vi "Main.vi"() -> ()   [LabVIEW 2025]
panel:
  out "Available Cash":dbl
  out "Password Exist?":bool
  in  "Input":string
  in  "Exit":bool
  in  "Fast Cash (50)":bool
  in  "Deposit":bool
  in  "Withdraw":bool
  in  "Login":bool
  out "ATM window":string
  in  "Tab Control":enum32{"ATM"}(tab)
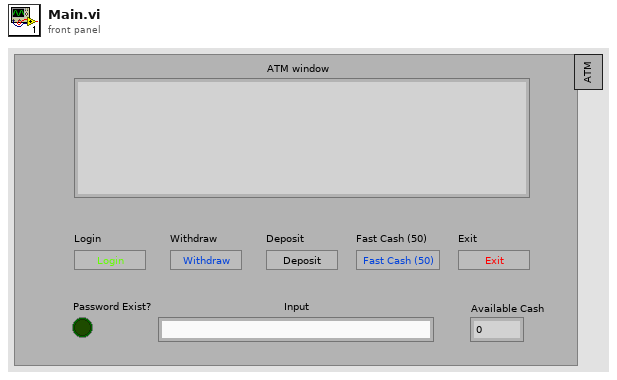
[diagram p1: front panel]
types:
  T1 = cluster{"Data":string[][], "User_ID":i32, "Password Exist?":bool, "ATM window":string, "Cash":dbl}
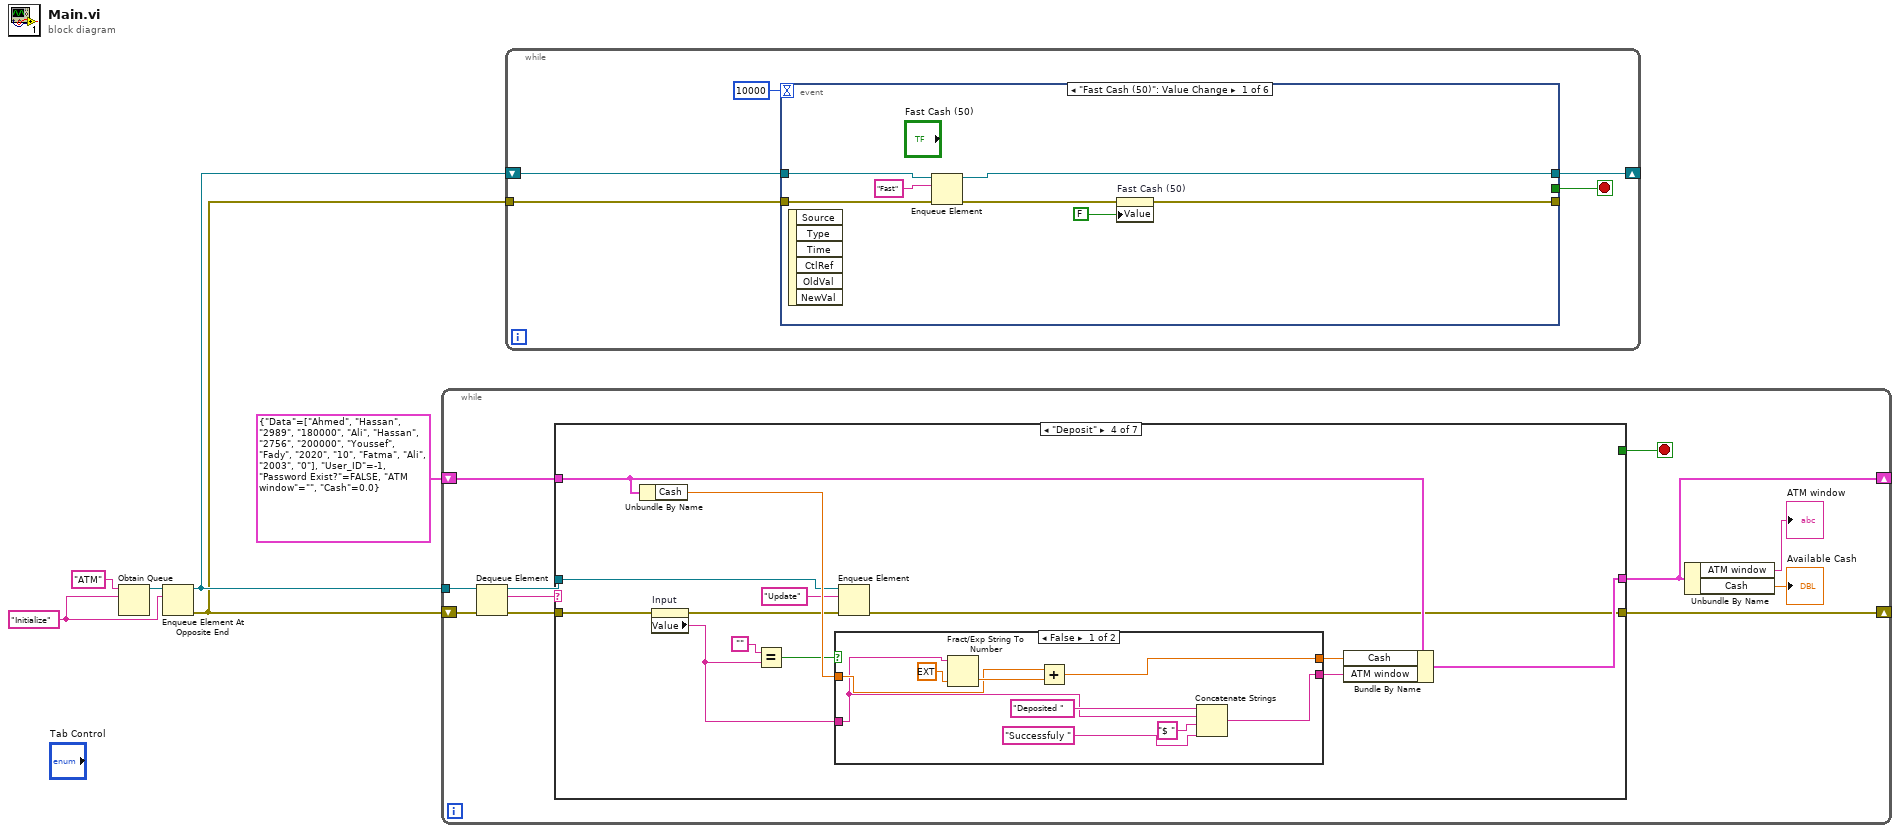
[diagram p0: block diagram]
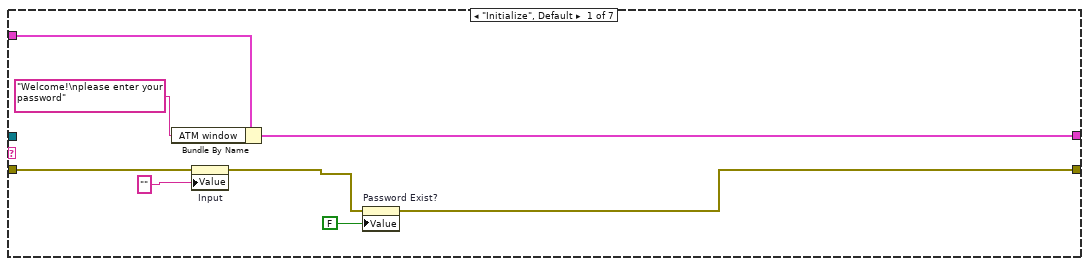
[diagram p2: hidden frame]
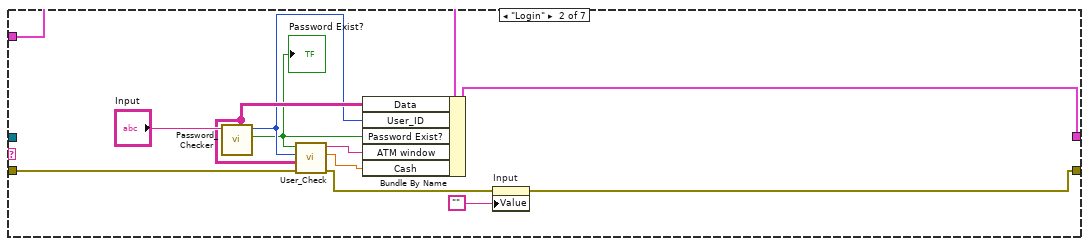
[diagram p3: hidden frame]
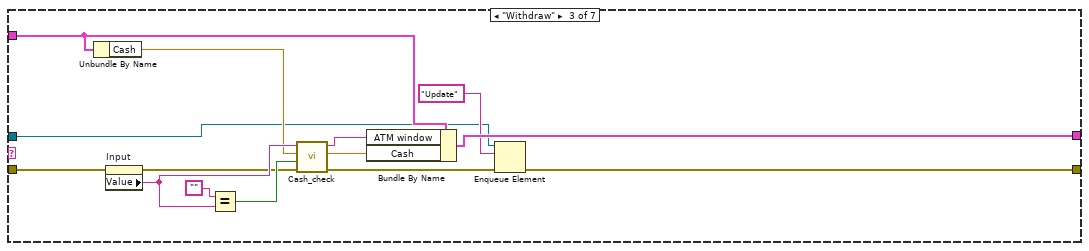
[diagram p4: hidden frame]
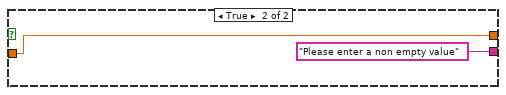
[diagram p5: hidden frame]
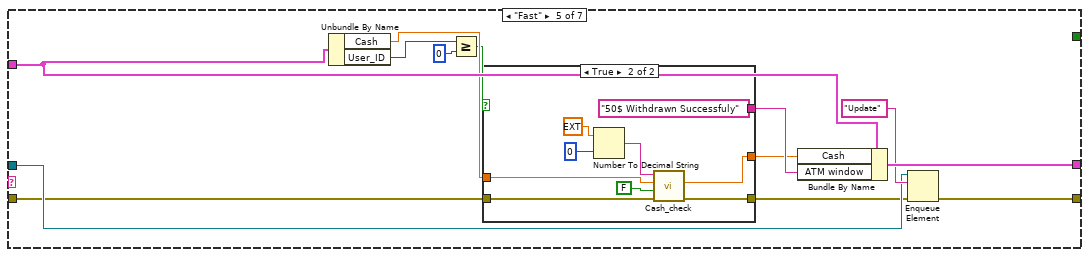
[diagram p6: hidden frame]
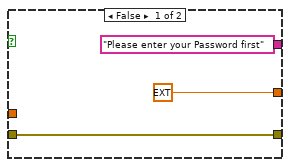
[diagram p7: hidden frame]
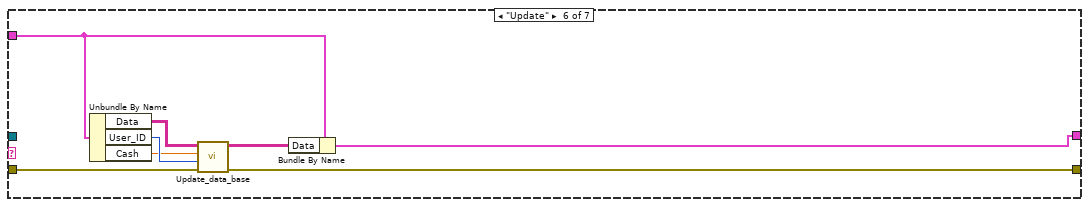
[diagram p8: hidden frame]
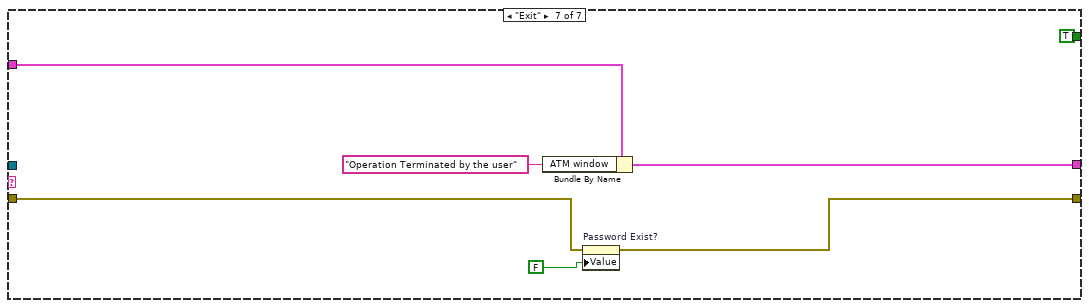
[diagram p9: hidden frame]
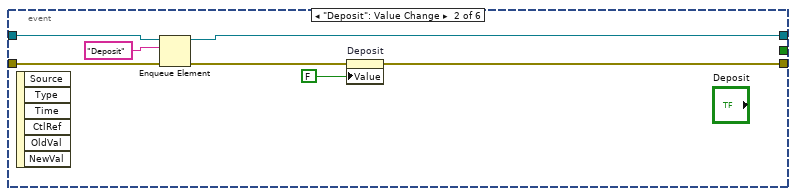
[diagram p10: hidden frame]
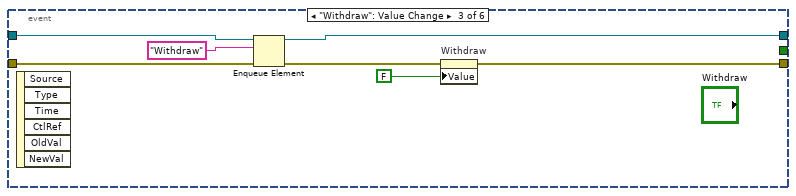
[diagram p11: hidden frame]
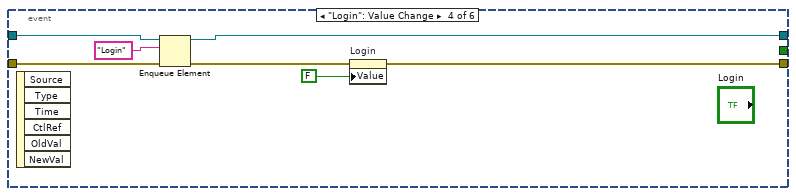
[diagram p12: hidden frame]
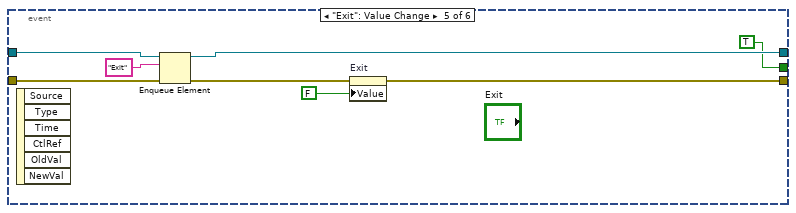
[diagram p13: hidden frame]
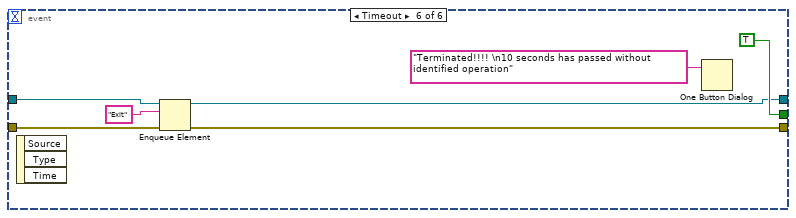
[diagram p14: hidden frame]
diagram:
  w4 = "Initialize" ("element")
  n1 = Obtain Queue(name (unnamed)="ATM", element data type=w4) -> (queue out=w5:refnum<queue>)  [unwired: 3 in, 2 out]
  n2 = Enqueue Element At Opposite End(queue=w5, element=w4) -> (queue out=w3:refnum<queue>, error out=w2:errorcluster)  [unwired: 2 in, 1 out]
  n3 = while {
    tunnel: w3 -> [w17]
    shift-right: [w9] -> _
    shift-left: T1 {"Data"=[["Ahmed", "Hassan", "2989", "180000"], ["Ali", "Hassan", "2756", "200000"], ["Youssef", "Fady", "2020", "10"], ["Fatma", "Ali", "2003", "0"]], "User_ID"=-1, "Password Exist?"=FALSE, "ATM window"="", "Cash"=0.0} -> [w12]
    shift-right: [w10] -> _
    shift-left: w2 -> [w16]
    stop <- w7 stop-if-true
    n4 = Dequeue Element(queue=w17, error in (no error)=w16) -> (queue out=w13:refnum<queue>, element=w15:string, error out=w14:errorcluster)  [unwired: 1 in, 1 out]
    n5 = case shown="\"Deposit\"" w15 {
      tunnel: w14 -> [w22 w36 w50 w64 w81 w108 w111]
      tunnel: w13 -> [_ _ w38 w58 w84 _ _]
      tunnel: [w23 w30 w42 w60 w86 w101 w112] -> w9
      tunnel: w12 -> [w25 w35 w45 w62 w88 w103 w114]
      tunnel: [w18 w27 w39 w56 w83 w107 w109] -> w10
      tunnel: [_ _ _ _ _ _ TRUE ("stop 2")] -> w7
      frame "Initialize", Default {
        n6 = Bundle By Name(cluster=w25, "ATM window"="Welcome!\nplease enter your password" ("element")) -> (w23:T1)
        n7 = property on="Input" class="Str"(error in=w22, "Value"="" ("Input")) -> (error out=w19:errorcluster)  [unwired: 1 in, 1 out]
        n8 = property on="Password Exist?" class="Bool (strict)"(error in=w19, "Value"=FALSE ("Password Exist?")) -> (error out=w18:errorcluster)  [unwired: 1 in, 1 out]
      }
      frame "Login" {
        n9 = call "Password_Checker.vi"("Password"="Input") -> ("Password Exist?"=w32:bool, "User_ID"=w33:i32, "Data"=w34:string[][])  [unwired: 7 in, 1 out]
        "Password Exist?" <- w32
        n10 = call "User_Check.vi"("error in (no error)"=w36, "Array"=w34, "User_id"=w33, "User found"=w32) -> ("error out"=w28:errorcluster, "Cash"=w29:dbl, "ATM window"=w31:string)  [unwired: 5 in]
        n11 = Bundle By Name(cluster=w35, "Data"=w34, "User_ID"=w33, "Password Exist?"=w32, "ATM window"=w31, "Cash"=w29) -> (w30:T1)
        n12 = property on="Input" class="Str"(error in=w28, "Value"="") -> (error out=w27:errorcluster)  [unwired: 1 in, 1 out]
      }
      frame "Withdraw" {
        n13 = Unbundle By Name(w45) -> ("Cash"=w47:dbl)
        n14 = property on="Input" class="Str"(error in=w50) -> (error out=w46:errorcluster, "Value"=w48:string)  [unwired: 1 in, 1 out]
        n15 = Equal?(x="", y=w48) -> (x = y?=w49:bool)
        n16 = call "Cash_check.vi"("error in (no error)"=w46, "Empty"=w49, "cash"=w47, "input"=w48) -> ("error out"=w40:errorcluster, "new cash"=w43:ext, "ATM window"=w44:string)  [unwired: 5 in]
        n17 = Bundle By Name(cluster=w45, "ATM window"=w44, "Cash"=w43) -> (w42:T1)
        n18 = Enqueue Element(queue=w38, element="Update", error in (no error)=w40) -> (error out=w39:errorcluster)  [unwired: 1 in, 2 out]
      }
      frame "Deposit" {
        n19 = Unbundle By Name(w62) -> ("Cash"=w63:dbl)
        n20 = property on="Input" class="Str"(error in=w64) -> (error out=w57:errorcluster, "Value"=w53:string)  [unwired: 1 in, 1 out]
        n21 = Equal?(x="", y=w53) -> (x = y?=w52:bool)
        n22 = case shown="False" w52 {
          tunnel: w63 -> [w71 w75]
          tunnel: [w70 w75] -> w61
          tunnel: [w67 "Please enter a non empty value"] -> w55
          tunnel: w53 -> [w65 _]
          frame False {
            n23 = Fract/Exp String To Number(string=w65, default (0 dbl)=ext 0.0 ("default (0 DBL)")) -> (number=w72:ext)  [unwired: 2 in, 1 out]
            n24 = Add(x=w71, y=w72) -> (x+y=w70:ext)
            n25 = Concatenate Strings("Deposited " ("ATM window"), w65, "$ " ("string"), "Successfuly " ("ATM window")) -> (w67:string)
          }
          frame True {
          }
        }
        n26 = Enqueue Element(queue=w58, element="Update", error in (no error)=w57) -> (error out=w56:errorcluster)  [unwired: 1 in, 2 out]
        n27 = Bundle By Name(cluster=w62, "Cash"=w61, "ATM window"=w55) -> (w60:T1)
      }
      frame "Fast" {
        n28 = Unbundle By Name(w88) -> ("Cash"=w82:dbl, "User_ID"=w77:i32)
        n29 = Greater Or Equal?(x=w77, y=0) -> (x >= y?=w76:bool)
        n30 = case shown="True" w76 {
          tunnel: ["Please enter your Password first" ("ATM window") "50$ Withdrawn Successfuly" ("ATM window")] -> w87
          tunnel: w82 -> [_ w99]
          tunnel: w81 -> [w89 w94]
          tunnel: [w89 w93] -> w80
          tunnel: [ext 0.0 ("new cash") w92] -> w79
          frame False {
          }
          frame True {
            n31 = Number To Decimal String(number=ext 50.0 ("default (0 DBL)"), width (-)=i16 0) -> (decimal integer string=w96:string)
            n32 = call "Cash_check.vi"("error in (no error)"=w94, "Empty"=FALSE, "cash"=w99, "input"=w96) -> ("error out"=w93:errorcluster, "new cash"=w92:ext)  [unwired: 5 in, 1 out]
          }
        }
        n33 = Bundle By Name(cluster=w88, "Cash"=w79, "ATM window"=w87) -> (w86:T1)
        n34 = Enqueue Element(queue=w84, element="Update", error in (no error)=w80) -> (error out=w83:errorcluster)  [unwired: 1 in, 2 out]
      }
      frame "Update" {
        n35 = Unbundle By Name(w103) -> ("Data"=w106:string[][], "User_ID"=w105:i32, "Cash"=w104:dbl)
        n36 = call "Update_data_base.vi"("error in (no error)"=w108, "User id"=w105, "Cach"=w104, "Data base"=w106) -> ("error out"=w107:errorcluster, "New Data Base"=w102:string[][])  [unwired: 6 in]
        n37 = Bundle By Name(cluster=w103, "Data"=w102) -> (w101:T1)
      }
      frame "Exit" {
        n38 = Bundle By Name(cluster=w114, "ATM window"="Operation Terminated by the user") -> (w112:T1)
        n39 = property on="Password Exist?" class="Bool (strict)"(error in=w111, "Value"=FALSE ("Password Exist?")) -> (error out=w109:errorcluster)  [unwired: 1 in, 1 out]
      }
    }
    n40 = Unbundle By Name(w9) -> ("ATM window"=→"ATM window":string, "Cash"=→"Available Cash":dbl)
  }
  n41 = while {
    shift-right: [w119] -> _
    shift-left: w3 -> [w120]
    tunnel: w2 -> [w118]
    stop <- w116 stop-if-true
    n42 = event shown="[0] \"Fast Cash (50)\": Value Change" {
      selector: _ -> [_ _ _ _ _ _]
      dyn-events: _ -> [_ _ _ _ _ _]
      timeout: 10000 -> [_ _ _ _ _ _]
      tunnel: w120 -> [w126 w133 w140 w148 w154 w161]
      tunnel: [w125 w131 w139 w146 w153 w158] -> w119
      tunnel: w118 -> [w124 w132 w138 w144 w156 w160]
      tunnel: [w122 w128 w135 w142 w149 w159] -> _
      tunnel: [_ _ _ _ TRUE ("stop") TRUE ("stop")] -> w116
      event "Fast Cash (50)": Value Change {
        n43 = event-data() -> ()  [unwired: 1 in, 6 out]
        n44 = Enqueue Element(queue=w126, element="Fast", error in (no error)=w124) -> (queue out=w125:refnum<queue>, error out=w123:errorcluster)  [unwired: 1 in, 1 out]
        n45 = property on="Fast Cash (50)" class="Bool (strict)"(error in=w123, "Value"=FALSE ("Fast Cash (50)")) -> (error out=w122:errorcluster)  [unwired: 1 in, 1 out]
      }
      event "Deposit": Value Change {
        n46 = event-data() -> ()  [unwired: 1 in, 6 out]
        n47 = Enqueue Element(queue=w133, element="Deposit", error in (no error)=w132) -> (queue out=w131:refnum<queue>, error out=w129:errorcluster)  [unwired: 1 in, 1 out]
        n48 = property on="Deposit" class="Bool (strict)"(error in=w129, "Value"=FALSE ("Deposit")) -> (error out=w128:errorcluster)  [unwired: 1 in, 1 out]
      }
      event "Withdraw": Value Change {
        n49 = event-data() -> ()  [unwired: 1 in, 6 out]
        n50 = Enqueue Element(queue=w140, element="Withdraw", error in (no error)=w138) -> (queue out=w139:refnum<queue>, error out=w136:errorcluster)  [unwired: 1 in, 1 out]
        n51 = property on="Withdraw" class="Bool (strict)"(error in=w136, "Value"=FALSE ("Withdraw")) -> (error out=w135:errorcluster)  [unwired: 1 in, 1 out]
      }
      event "Login": Value Change {
        n52 = event-data() -> ()  [unwired: 1 in, 6 out]
        n53 = Enqueue Element(queue=w148, element="Login", error in (no error)=w144) -> (queue out=w146:refnum<queue>, error out=w143:errorcluster)  [unwired: 1 in, 1 out]
        n54 = property on="Login" class="Bool (strict)"(error in=w143, "Value"=FALSE ("Login")) -> (error out=w142:errorcluster)  [unwired: 1 in, 1 out]
      }
      event "Exit": Value Change {
        n55 = event-data() -> ()  [unwired: 1 in, 6 out]
        n56 = Enqueue Element(queue=w154, element="Exit", error in (no error)=w156) -> (queue out=w153:refnum<queue>, error out=w151:errorcluster)  [unwired: 1 in, 1 out]
        n57 = property on="Exit" class="Bool (strict)"(error in=w151, "Value"=FALSE ("Exit")) -> (error out=w149:errorcluster)  [unwired: 1 in, 1 out]
      }
      event Timeout {
        n58 = event-data() -> ()  [unwired: 1 in, 3 out]
        n59 = Enqueue Element(queue=w161, element="Exit", error in (no error)=w160) -> (queue out=w158:refnum<queue>, error out=w159:errorcluster)  [unwired: 1 in, 1 out]
        n60 = One Button Dialog(message="Terminated!!!! \n10 seconds has passed without identified operation") -> ()  [unwired: 1 in, 1 out]
      }
    }
  }
